vi "Set_CHROMA.vi"(3 "instrument handle out":refnum<k15>) -> (11 "instrument handle":refnum<k15>)   [LabVIEW 2014]
uses:
  FT_HMI.llb/GLOBAL_GEN.vi
  FT_HMI.llb/GLOBAL_PUMPS_PARAMS.vi
panel:
  in  "instrument handle out 2":refnum<k15>
  out "instrument handle 2":refnum<k15>
  out "id string":string
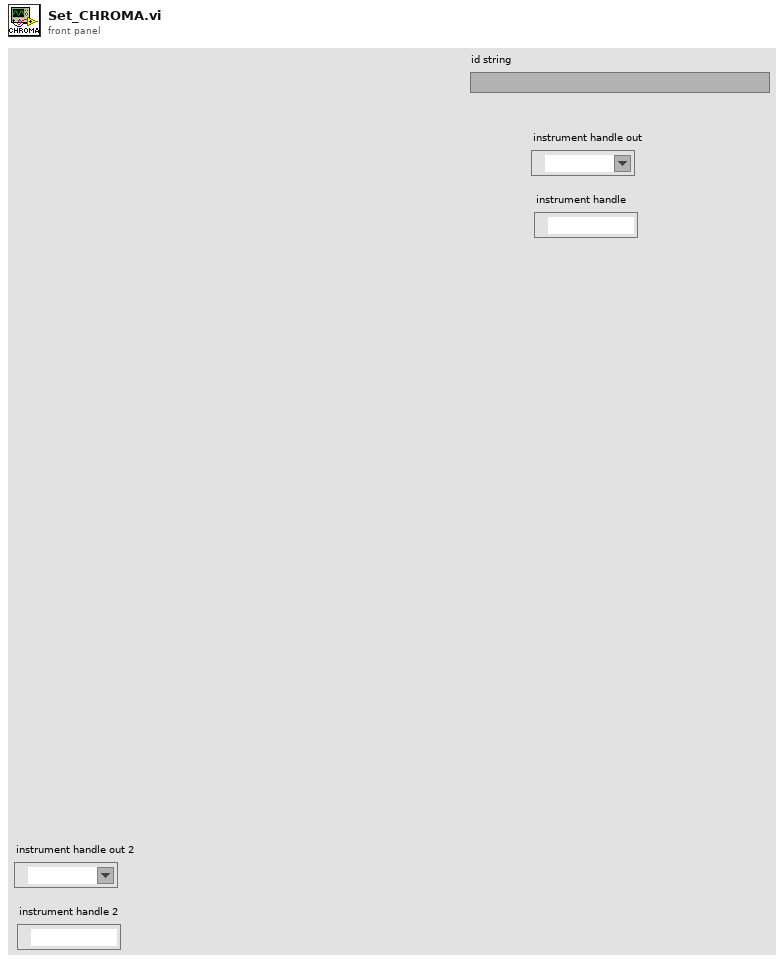
[diagram p1: front panel]
types:
  T1 = cluster{"GENERAL":cluster{"NO ARTICLE":string, "DESIGNATION":string, "TENSION [V]":sgl, "FREQUENCE [Hz]":sgl, "BYPASS":bool}, "ST1_HT":cluster{"STATUS HT":bool, "TENSION ISOLATION [V]":sgl, "COURANT ISOLATION [mA]":sgl, "TEMPS DE MESURE [ms]":i32, "NO PROGRAMME":i32}, "ST2_ASPIRATION":cluster{"STATUS H ASP":bool, "TEMPS POMPAGE [ms]":i32, "STATUS CONTRE-PRESSION":bool, "HAUTEUR ASPIRATION [m]":sgl, "TEMPS DE MESURE ASP [ms]":i32, "STATUS PERTE ASP":bool, "PERTE ASPIRATION [mbar]":sgl, "TEMPS DE MESURE PERTE [ms] ":i32}, "ST3_ETANCHEITE":cluster{"STATUS":bool, "ETANCHEITE [mbar]":sgl, "TEMPS MISE SOUS PRESSION [ms]":i32, "TEMPS STABILISATION [ms]":i32, "TEMPS DE MESURE [ms]":i32}, "ST4-5_DEBIT":cluster{"STATUS QMAX":bool, "GRAND DEBIT":bool, "PUMPING_TIME  [ms]":i32, "DEBIT MIN [l/h]":sgl, "DEBIT MAX  [l/h]":sgl, "TEMPS DE MESURE QMAX [ms]":i32, "STATUS QTRAVAIL 1":bool, "DEBIT TRAVAIL 1 MIN [l/h]":sgl, "DEBIT TRAVAIL 1 MAX [l/h]":sgl, "PRESSION DE CONSIGNE 1 [bar]":sgl, "TEMPS DE REGLAGE PRESSION [ms]":i32, "TEMPS DE MESURE QTRAVAIL 1 [ms]":i32, "STATUS QTRAVAIL 2":bool, "DEBIT TRAVAIL 2 MIN [l/h]":sgl, "DEBIT TRAVAIL 2 MAX [l/h]":sgl, "PRESSION DE CONSIGNE 2 [bar]":sgl, "TEMPS DE MESURE QTRAVAIL 2 [ms]":i32, "STATUS CONSO":bool, "CONSOMMATION [A]":sgl, "TEMPS DE MESURE COURANT [ms]":i32}, "ST6_PRESSION":cluster{"STATUS PMAX":bool, "PUMPING TIME [ms]":i32, "PRESSION MIN [bar]":sgl, "TEMPS DE MESURE PMAX [ms]":i32, "STATUS PERTE PRESSION":bool, "PERTE PRESSION [mbar]":sgl, "TEMPS DE MESURE PERTE [ms]":i32}, "ST7_VIDANGE":cluster{"STATUS VIDANGE":bool, "TEMPS DE VIDANGE [ms] ":i32}, "ST8_IMPRESSION":cluster{"STATUS":bool, "ETIQUETTE":string}, "ST9_DECHARGEMENT":cluster{"STATUS":bool, "BOBINE A FIL":bool}, "DIVERS":cluster{"INDICE MODIF":string, "DATE MODIF":timestamp, "HISTORIQUE MODIF":string, "EMBOUT PRESSION":string, "EMBOUT ASPIRATION":string}}
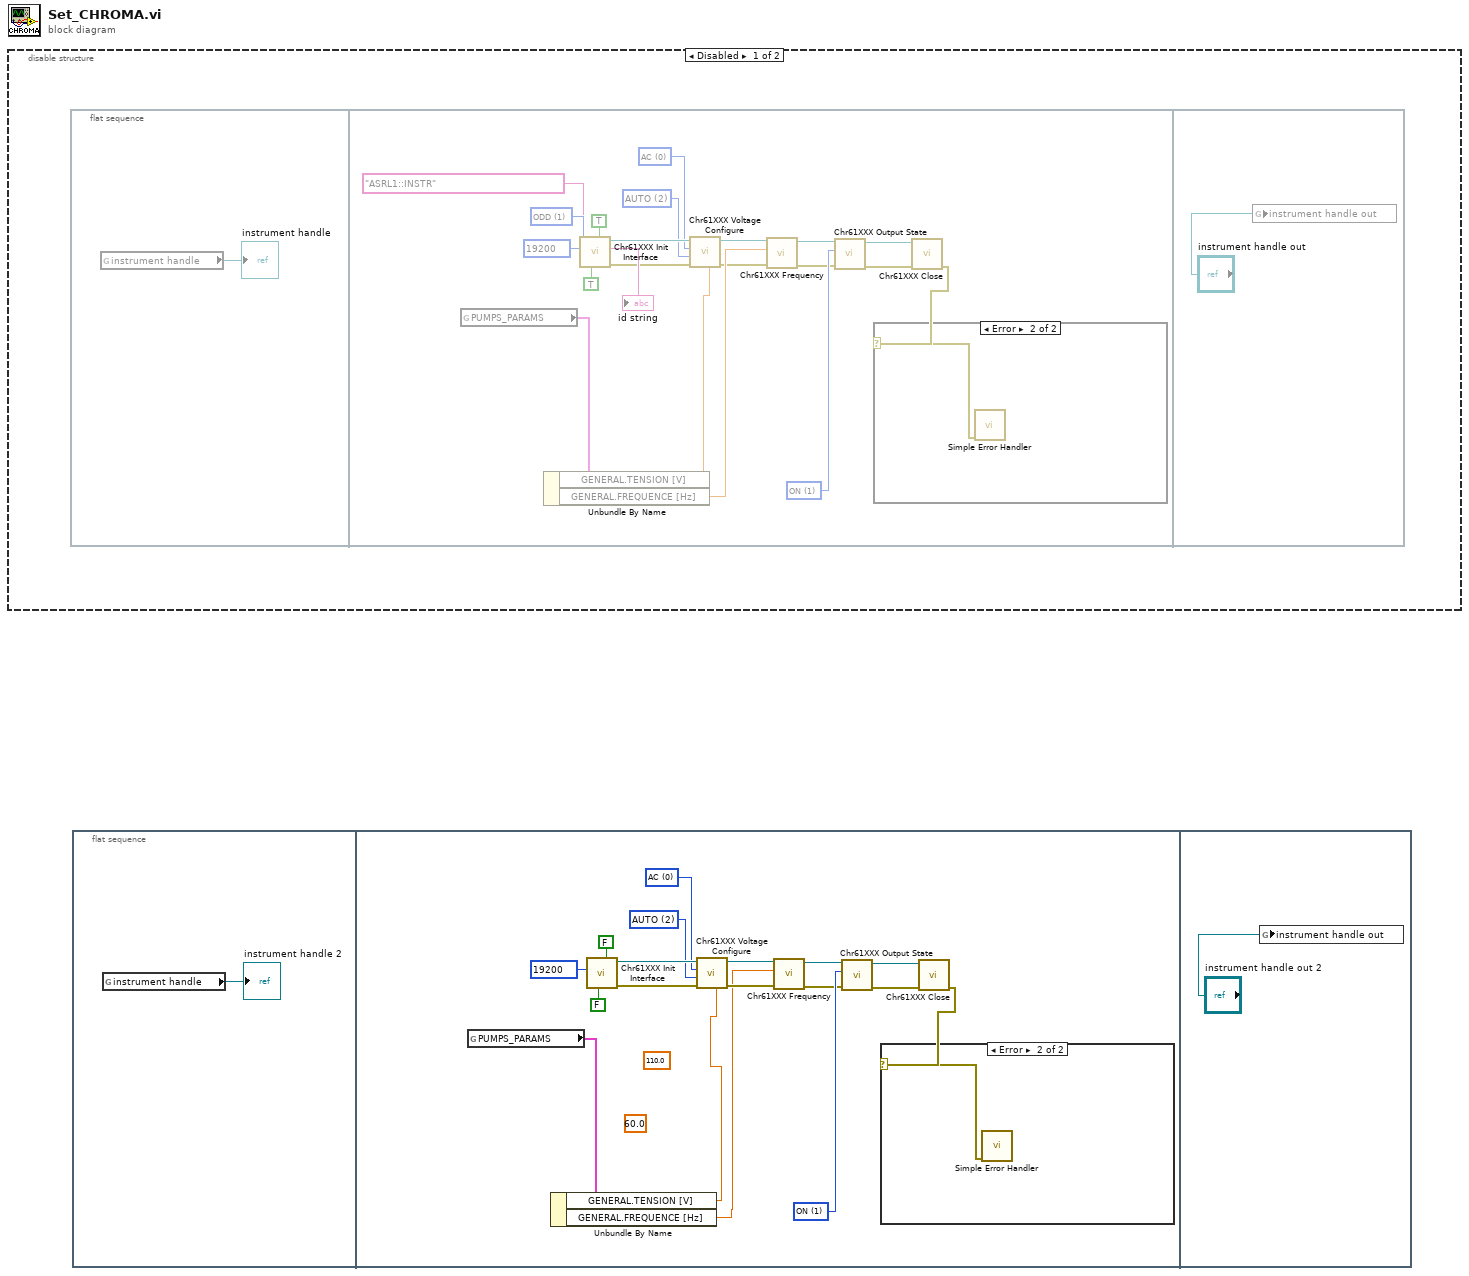
[diagram p0: block diagram]
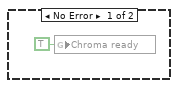
[diagram p2: hidden frame]
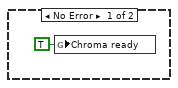
[diagram p4: hidden frame]
diagram:
  n1 = disable-structure shown="Disabled" {
    frame Disabled {
      n2 = flat-sequence {
        frame #0 {
          n3 = global read "GLOBAL_GEN.vi" "instrument handle"() -> (→"instrument handle":refnum<k15>)
        }
        frame #1 {
          w9 = 1 items=["NONE", "ODD", "EVEN"] ("parity")
          w15 = 19200 items=["9600"=9600, "19200"=19200, "38400"=38400, "57600"=57600, "115200"=115200] ("baud rate")
          w20 = 2 items=["LOW", "HIGH", "AUTO"] ("voltage range")
          w19 = 0 items=["AC", "DC"] ("voltage type")
          w16 = u16 1 items=["OFF", "ON"] ("state")
          n4 = global read "GLOBAL_PUMPS_PARAMS.vi" "PUMPS_PARAMS"() -> (w12:T1)
          n5 = Unbundle By Name(w12) -> ("GENERAL.TENSION [V]"=w11:sgl, "GENERAL.FREQUENCE [Hz]"=w10:sgl)
          n6 = call <instrlib>:"Chr61XXX Init Interface.vi"("id query"=TRUE, "reset device"=TRUE, "parity"=w9, "baud rate"=w15, "resource name"="ASRL1::INSTR") -> ("error out"=w6:errorcluster, "id string"=→"id string":string, "instrument handle out"=w21:refnum<k15>)  [unwired: 4 in]
          n7 = call <instrlib>:"Chr61XXX Voltage Configure.vi"("voltage"=w11, "error in (no error)"=w6, "voltage range"=w20, "voltage type"=w19, "instrument handle"=w21) -> ("error out"=w5:errorcluster, "instrument handle out"=w18:refnum<k15>)  [unwired: 5 in]
          n8 = call <instrlib>:"Chr61XXX Frequency.vi"("error in (no error)"=w5, "frequency"=w10, "instrument handle"=w18) -> ("error out"=w4:errorcluster, "instrument handle out"=w17:refnum<k15>)  [unwired: 7 in]
          n9 = call <instrlib>:"Chr61XXX Output State.vi"("error in (no error)"=w4, "state"=w16, "instrument handle"=w17) -> ("error out"=w3:errorcluster, "instrument handle out"=w22:refnum<k15>)  [unwired: 7 in]
          n10 = call <instrlib>:"Chr61XXX Close.vi"("error in (no error)"=w3, "instrument handle"=w22) -> ("error out"=w7:errorcluster)  [unwired: 9 in]
          n11 = case shown="Error" w7 {
            selector: w7 -> [_ w24]
            frame No Error {
              n12 = global write "GLOBAL_GEN.vi" "Chroma ready"(TRUE ("Chroma ready")) -> ()
            }
            frame Error {
              n13 = call <vilib>:"Simple Error Handler.vi"("error in (no error)"=w24) -> ()  [unwired: 4 in, 5 out]
            }
          }
        }
        frame #2 {
          n14 = global write "GLOBAL_GEN.vi" "instrument handle out"("instrument handle out") -> ()
        }
      }
    }
    frame Enabled {
    }
  }
  n15 = flat-sequence {
    frame #0 {
      n16 = global read "GLOBAL_GEN.vi" "instrument handle"() -> (→"instrument handle 2":refnum<k15>)
    }
    frame #1 {
      (unwired) 60.0
      (unwired) 110.0
      w37 = 19200 items=["9600"=9600, "19200"=19200, "38400"=38400, "57600"=57600, "115200"=115200] ("baud rate")
      w42 = 2 items=["LOW", "HIGH", "AUTO"] ("voltage range")
      w41 = 0 items=["AC", "DC"] ("voltage type")
      w38 = u16 1 items=["OFF", "ON"] ("state")
      n17 = global read "GLOBAL_PUMPS_PARAMS.vi" "PUMPS_PARAMS"() -> (w34:T1)
      n18 = Unbundle By Name(w34) -> ("GENERAL.TENSION [V]"=w28:sgl, "GENERAL.FREQUENCE [Hz]"=w27:sgl)
      n19 = call <instrlib>:"Chr61XXX Init Interface.vi"("id query"=FALSE, "reset device"=FALSE, "baud rate"=w37) -> ("error out"=w32:errorcluster, "instrument handle out"=w43:refnum<k15>)  [unwired: 6 in, 1 out]
      n20 = call <instrlib>:"Chr61XXX Voltage Configure.vi"("voltage"=w28, "error in (no error)"=w32, "voltage range"=w42, "voltage type"=w41, "instrument handle"=w43) -> ("error out"=w31:errorcluster, "instrument handle out"=w40:refnum<k15>)  [unwired: 5 in]
      n21 = call <instrlib>:"Chr61XXX Frequency.vi"("error in (no error)"=w31, "frequency"=w27, "instrument handle"=w40) -> ("error out"=w30:errorcluster, "instrument handle out"=w39:refnum<k15>)  [unwired: 7 in]
      n22 = call <instrlib>:"Chr61XXX Output State.vi"("error in (no error)"=w30, "state"=w38, "instrument handle"=w39) -> ("error out"=w29:errorcluster, "instrument handle out"=w44:refnum<k15>)  [unwired: 7 in]
      n23 = call <instrlib>:"Chr61XXX Close.vi"("error in (no error)"=w29, "instrument handle"=w44) -> ("error out"=w33:errorcluster)  [unwired: 9 in]
      n24 = case shown="Error" w33 {
        selector: w33 -> [_ w46]
        frame No Error {
          n25 = global write "GLOBAL_GEN.vi" "Chroma ready"(TRUE ("Chroma ready")) -> ()
        }
        frame Error {
          n26 = call <vilib>:"Simple Error Handler.vi"("error in (no error)"=w46) -> ()  [unwired: 4 in, 5 out]
        }
      }
    }
    frame #2 {
      n27 = global write "GLOBAL_GEN.vi" "instrument handle out"("instrument handle out 2") -> ()
    }
  }
